vi "Connection Database.vi"(8 "error in (no error)":errorcluster caption="错误输入（无错误）", 11 "Connncet State":T1) -> (0 "error out":errorcluster caption="错误输出", 3 "Connncet State out":T1)   [LabVIEW 2014]
uses:
  <vilib>/addons/database/NI_Database_API.lvlib
  <vilib>/addons/database/Connection.llb/DB Tools Open Connec (String).vi
  Ctr/Constr.ctl
  <vilib>/addons/database/Connection.llb/Conn ObjectReference.ctl
  Ctr/Conneect State.ctl
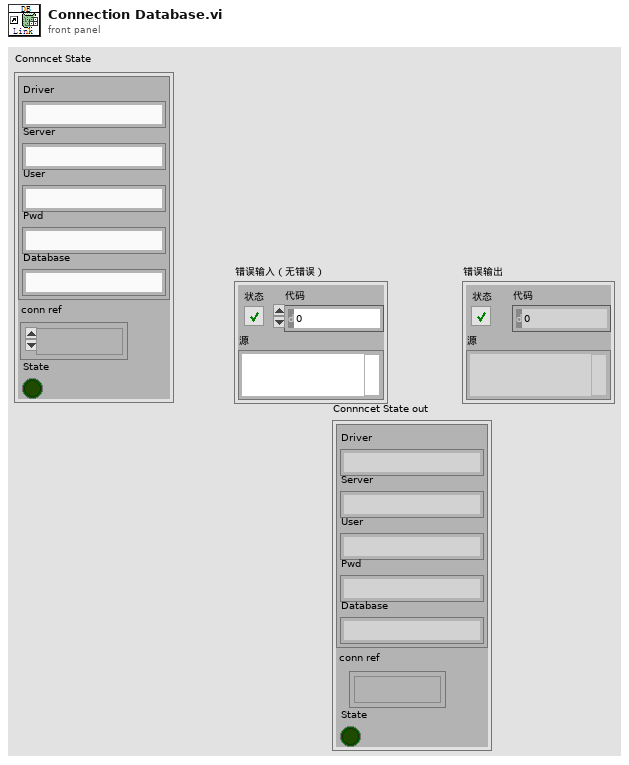
[diagram p1: front panel]
types:
  T1 = typedef "Conneect State.ctl" = cluster{"Constr":T2, "conn ref":T3, "State":bool}
  T2 = typedef "Constr.ctl" = cluster{"Driver":string, "Server":string, "User":string, "Pwd":string, "Database":string}
  T3 = typedef "NI_Database_API.lvlib/Conn ObjectReference.ctl" = refnum<k1>
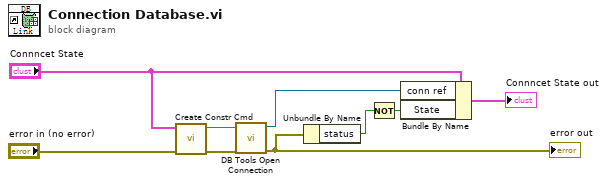
[diagram p0: block diagram]
diagram:
  n1 = call "Create Constr Cmd.vi"("error in (no error)"="error in (no error)", "Connncet State"="Connncet State") -> ("error out"=w5:errorcluster, "Constr"=w4:string)  [unwired: 8 in]
  n2 = call-poly <vilib>:"DB Tools Open Connection.vi"("error in (no error)"=w5, "connection information"=w4) -> ("error out"=w7:errorcluster, "connection reference"=w3:T3)  [unwired: 6 in]
  "error out" <- w7
  n3 = Unbundle By Name(w7) -> ("status"=w1:bool)
  n4 = Not(x=w1) -> (.not. x?=w2:bool)
  n5 = Bundle By Name(cluster="Connncet State", "conn ref"=w3, "State"=w2) -> (→"Connncet State out":T1)
